vi "Command - ERROR (SubVI) - C.vi"(0 "ESP Config":T1={"COM Port Input"="COM8", "Manual Command"={"Device Type"="", "Instance"="", "Command"="", "Sub-Command"="", "Parameters (Seperate by :)"=""}, "Device Type"="e", "Instance"="a", "Use Manual Command"=FALSE, "Timeout [msec]"=1000, "Read/Write Wait [msec]"=50}, 5 "ESP Table Cluster Ref":refnum<vi>, 7 "Display Cluster Ref":refnum<vi>) -> (10 "ERROR Data":string, 15 "ERROR List":errorcluster)   [LabVIEW 2011]
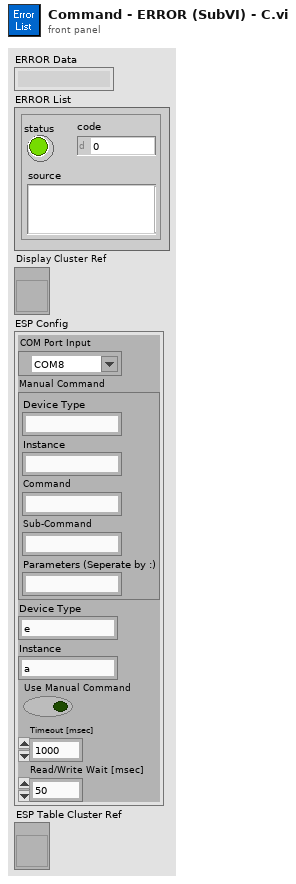
[diagram p1: front panel]
types:
  T1 = cluster{"COM Port Input":refnum<visa-resource-name>, "Manual Command":cluster{"Device Type":string, "Instance":string, "Command":string, "Sub-Command":string, "Parameters (Seperate by :)":string}, "Device Type":string, "Instance":string, "Use Manual Command":bool, "Timeout [msec]":u32, "Read/Write Wait [msec]":u32}
  T2 = cluster{"ON Demand Button":i32, "ON Demand Commands":i32, "Continuous Button":i32, "Continuous Commands":i32, "Error Button":i32, "Error Command":i32, "Status Button":i32, "Status Command":i32, "Digital Button":i32, "Digital Command":i32, "Save Table Button":i32, "Active Table":i32, "New Table Name":i32, "Table":i32}
  T3 = cluster{"Device Type":string, "Instance":string, "Command":string, "Sub-Command":string, "Parameters (Seperate by :)":string}
  T4 = cluster{"Write Command":string, "Read String":string, "Read Bytes":u32, "Bytes at Port":u32, "Response":string, "ACK":bool, "EOT":bool, "NAK":bool, "Parameters":string[]}
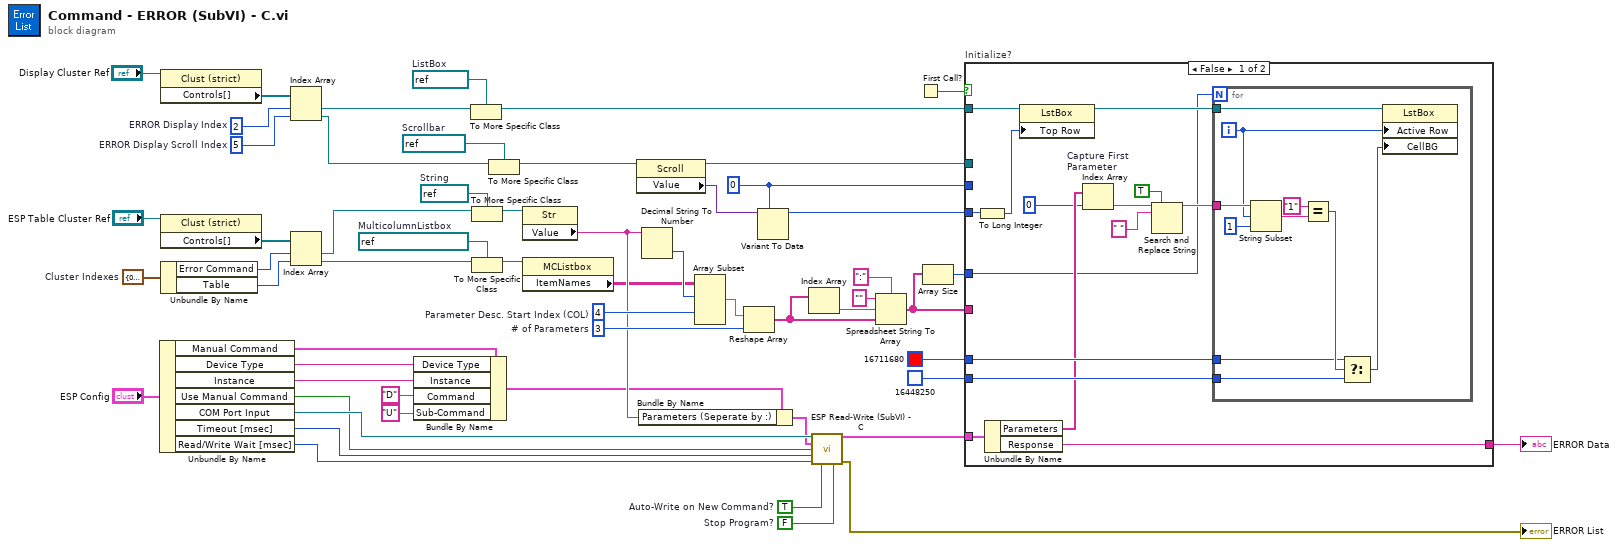
[diagram p0: block diagram]
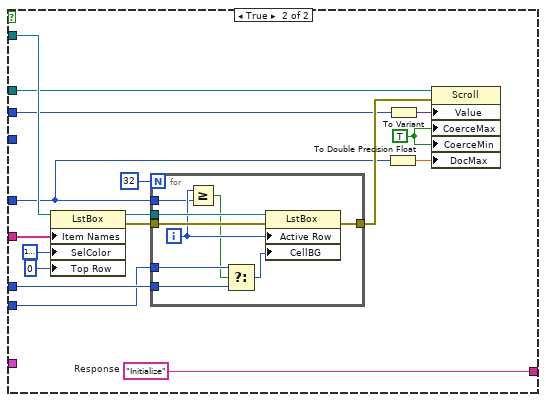
[diagram p2: hidden frame]
diagram:
  w9 = u8 0
  w15 = refnum<vi> refnum  # Scrollbar
  w17 = 5  # ERROR Display Scroll Index
  w18 = FALSE  # Stop Program?
  w19 = TRUE  # Auto-Write on New Command?
  w29 = refnum<vi> refnum  # ListBox
  w32 = 2  # ERROR Display Index
  w39 = T2 {"ON Demand Button"=0, "ON Demand Commands"=1, "Continuous Button"=2, "Continuous Commands"=3, "Error Button"=4, "Error Command"=5, "Status Button"=6, "Status Command"=7, "Digital Button"=8, "Digital Command"=9, "Save Table Button"=10, "Active Table"=11, "New Table Name"=12, "Table"=13}  # Cluster Indexes
  w42 = refnum<vi> refnum  # MulticolumnListbox
  w30 = refnum<vi> refnum  # String
  w51 = 3  # # of Parameters
  w52 = 4  # Parameter Desc. Start Index (COL)
  n1 = Unbundle By Name("ESP Config") -> ("Manual Command"=w45:T3, "Device Type"=w47:string, "Instance"=w46:string, "Use Manual Command"=w1:bool, "COM Port Input"=w25:refnum<visa-resource-name>, "Timeout [msec]"=w22:u32, "Read/Write Wait [msec]"=w21:u32)
  n2 = property class="Clust (strict)"(reference="Display Cluster Ref") -> ("Controls[]"=w33:refnum<vi>[])  [unwired: 1 in, 2 out]
  n3 = property class="Clust (strict)"(reference="ESP Table Cluster Ref") -> ("Controls[]"=w40:refnum<vi>[])  [unwired: 1 in, 2 out]
  n4 = Unbundle By Name(w39) -> ("Error Command"=w38:i32, "Table"=w37:i32)
  n5 = Index Array(array=w33, index #1=w32, index #2=w17) -> (element #1=w31:refnum<vi>, element #2=w16:refnum<vi>)
  n6 = Index Array(array=w40, index #1=w38, index #2=w37) -> (element #1=w34:refnum<vi>, element #2=w36:refnum<vi>)
  n7 = Bundle By Name(cluster=w45, "Device Type"=w47, "Instance"=w46, "Command"="D", "Sub-Command"="U") -> (w2:T3)
  n8 = To More Specific Class(target class=w29, reference=w31) -> (specific class reference=w28:refnum<vi>)  [unwired: 1 in, 1 out]
  n9 = To More Specific Class(target class=w30, reference=w34) -> (specific class reference=w43:refnum<vi>)  [unwired: 1 in, 1 out]
  n10 = To More Specific Class(target class=w42, reference=w36) -> (specific class reference=w41:refnum<vi>)  [unwired: 1 in, 1 out]
  n11 = To More Specific Class(target class=w15, reference=w16) -> (specific class reference=w14:refnum<vi>)  [unwired: 1 in, 1 out]
  n12 = property class="Str"(reference=w43) -> ("Value"=w27:string)  [unwired: 1 in, 2 out]
  n13 = property class="MCListbox"(reference=w41) -> ("ItemNames"=w26:string[][])  [unwired: 1 in, 2 out]
  n14 = property class="Scroll"(reference=w14) -> (reference out=w10:refnum<vi>, "Value"=w13:variant)  [unwired: 1 in, 1 out]
  n15 = Bundle By Name(cluster=w2, "Parameters (Seperate by :)"=w27) -> (w24:T3)
  n16 = Decimal String To Number(string=w27) -> (number=w55:i32)  [unwired: 2 in, 1 out]
  n17 = Array Subset(array=w26, index (row)=w55, index (col)=w52) -> (w53:string[][])  [unwired: 2 in]
  n18 = Reshape Array(w53, w51) -> (w5:string[])
  n19 = Variant To Data(type=w9, Variant=w13) -> (data=w12:u8)  [unwired: 1 in, 1 out]
  n20 = Index Array(array=w5) -> (element=w6:string)  [unwired: 1 in]
  n21 = call "ESP Read-Write (SubVI) - C.vi"("COM Port Input"=w25, "Command Input"=w24, "Manual Write Command"=w1, "Timeout (ms)"=w22, "Write/Read Wait (ms)"=w21, "Auto-Write on New Command?"=w19, "Stop Program?"=w18) -> ("ESP Values"=w23:T4, "Error Output"=→"ERROR List":errorcluster)  [unwired: 7 in]
  n22 = Spreadsheet String To Array(delimiter (Tab)=":", format string="", spreadsheet string=w6, array type (2D Dbl)=w5) -> (array=w4:string[])
  n23 = First Call?() -> (First Call?: T/F=w57:bool)
  n24 = Array Size(array=w4) -> (size(s)=w3:i32)
  n25 = case "Initialize?" shown="False" w57 {
    tunnel: w28 -> [w62 w99]
    tunnel: u32 16711680 -> [w72 w98]
    tunnel: u32 16448250 -> [w71 w87]
    tunnel: w23 -> [w70 _]
    tunnel: [w63 w94] -> w44
    tunnel: w12 -> [w60 _]
    tunnel: w10 -> [_ w92]
    tunnel: w9 -> [_ w88]
    tunnel: w4 -> [_ w86]
    tunnel: w3 -> [w59 w84]
    frame False {
      n26 = To Long Integer(number=w60) -> (32bit integer=w58:i32)
      n27 = Unbundle By Name(w70) -> ("Parameters"=w69:string[], "Response"=w63:string)
      n28 = property class="LstBox"(reference=w62, "Top Row"=w58) -> (reference out=w61:refnum<vi>)  [unwired: 1 in, 1 out]
      n29 = Index Array "Capture First \nParameter"(array=w69, index=0) -> (element=w64:string)
      n30 = Search and Replace String(replace all?=TRUE ("replace all? (F)"), input string=w64, search string=" ") -> (result string=w65:string)  [unwired: 5 in, 3 out]
      n31 = for {
        N: w59 -> [_]
        tunnel: w65 -> [w81]
        tunnel: w61 -> [w77]
        tunnel: w72 -> [w74]
        tunnel: w71 -> [w73]
        i -> [w76]
        n32 = String Subset(string=w81, offset (0)=w76, length (rest)=1 ("length (rest)")) -> (substring=w80:string)
        n33 = Equal?(x="1", y=w80) -> (x = y?=w75:bool)
        n34 = Select(t=w74, s=w75, f=w73) -> (s? t:f=w78:u32)
        n35 = property class="LstBox"(reference=w77, "Active Row"=w76, "CellBG"=w78) -> ()  [unwired: 1 in, 2 out]
      }
    }
    frame True {
      w85 = TRUE
      w94 = "Initialize"  # Response
      n36 = property class="LstBox"(reference=w99, "Item Names"=w86, "SelColor"=u32 16777216, "Top Row"=0) -> (reference out=w97:refnum<vi>, error out=w96:errorcluster)  [unwired: 1 in]
      n37 = for {
        N: 32 -> [_]
        tunnel: w97 -> [w108]
        tunnel: w96 -> [w107]
        tunnel: w98 -> [w101]
        tunnel: [w106] -> w89
        tunnel: w84 -> [w104]
        tunnel: w87 -> [w103]
        i -> [w105]
        n38 = Greater Or Equal?(x=w105, y=w104) -> (x >= y?=w102:bool)
        n39 = Select(t=w103, s=w102, f=w101) -> (s? t:f=w100:u32)
        n40 = property class="LstBox"(reference=w108, error in=w107, "Active Row"=w105, "CellBG"=w100) -> (error out=w106:errorcluster)  [unwired: 1 out]
      }
      n41 = To Double Precision Float(number=w84) -> (double precision float=w83:dbl)
      n42 = To Variant(anything=w88) -> (Variant=w91:variant)
      n43 = property class="Scroll"(reference=w92, error in=w89, "Value"=w91, "CoerceMax"=w85, "CoerceMin"=w85, "DocMax"=w83) -> ()  [unwired: 2 out]
    }
  }
  "ERROR Data" <- w44
